vi "TimeAlign.vi"(8 "error in (no error)":errorcluster, 11 "AllData In":T1 {"FlukeData"."DataAnalysisArray"."TimeStamp" format="%^<%.3X\n%x>T"; "FlukeData"."ModelDataArray"."FREQUENCY" format="%#_6f"; "FlukeData"."ModelDataArray"."TimeStamp" format="%^<%.3X\n%x>T"; "FlukeData"."PMUDataArray"."FREQUENCY" format="%#_6f"; "FlukeData"."PMUDataArray"."TimeStamp" format="%^<%.3X\n%x>T"; "NISTData"."DataAnlysisArray"."Time" format="%.6f"; "NISTData"."DataAnlysisArray"."TimeStamp" format="%^<%.3X\n%x>T"; "NISTData"."DUTDataArray"."TimeStamp" format="%^<%.3X\n%x>T"; "NISTData"."DUTDataArray"."Time" format="%.6f"; "NISTData"."NIDataArray"."TimeStamp" format="%^<%.3X\n%x>T"; "NISTData"."NIDataArray"."Time" format="%.6f"}) -> (0 "error out":errorcluster, 3 "AllData Out":T1 {"FlukeData"."DataAnalysisArray"."TimeStamp" format="%^<%.3X\n%x>T"; "FlukeData"."ModelDataArray"."FREQUENCY" format="%#_6f"; "FlukeData"."ModelDataArray"."TimeStamp" format="%^<%.3X\n%x>T"; "FlukeData"."PMUDataArray"."FREQUENCY" format="%#_6f"; "FlukeData"."PMUDataArray"."TimeStamp" format="%^<%.3X\n%x>T"; "NISTData"."DataAnlysisArray"."Time" format="%.6f"; "NISTData"."DataAnlysisArray"."TimeStamp" format="%^<%.3X\n%x>T"; "NISTData"."DUTDataArray"."TimeStamp" format="%^<%.3X\n%x>T"; "NISTData"."DUTDataArray"."Time" format="%.6f"; "NISTData"."NIDataArray"."TimeStamp" format="%^<%.3X\n%x>T"; "NISTData"."NIDataArray"."Time" format="%.6f"})   [LabVIEW 2014]
uses:
  typedefs/Alldata.ctl
  typedefs/NISTData.ctl
  typedefs/NIDataArray.ctl
  typedefs/NIData.ctl
  typedefs/PhasorRectangular.ctl
  typedefs/DUTData.ctl
  typedefs/NICalcAnalysis.ctl
  typedefs/CalcPhasorError.ctl
  typedefs/PlotDataArrays.ctl
  typedefs/PmuRawDataCluster.ctl
  typedefs/CalcAnalysis.ctl
panel:
  out "Search":timestamp
  out "Next":timestamp
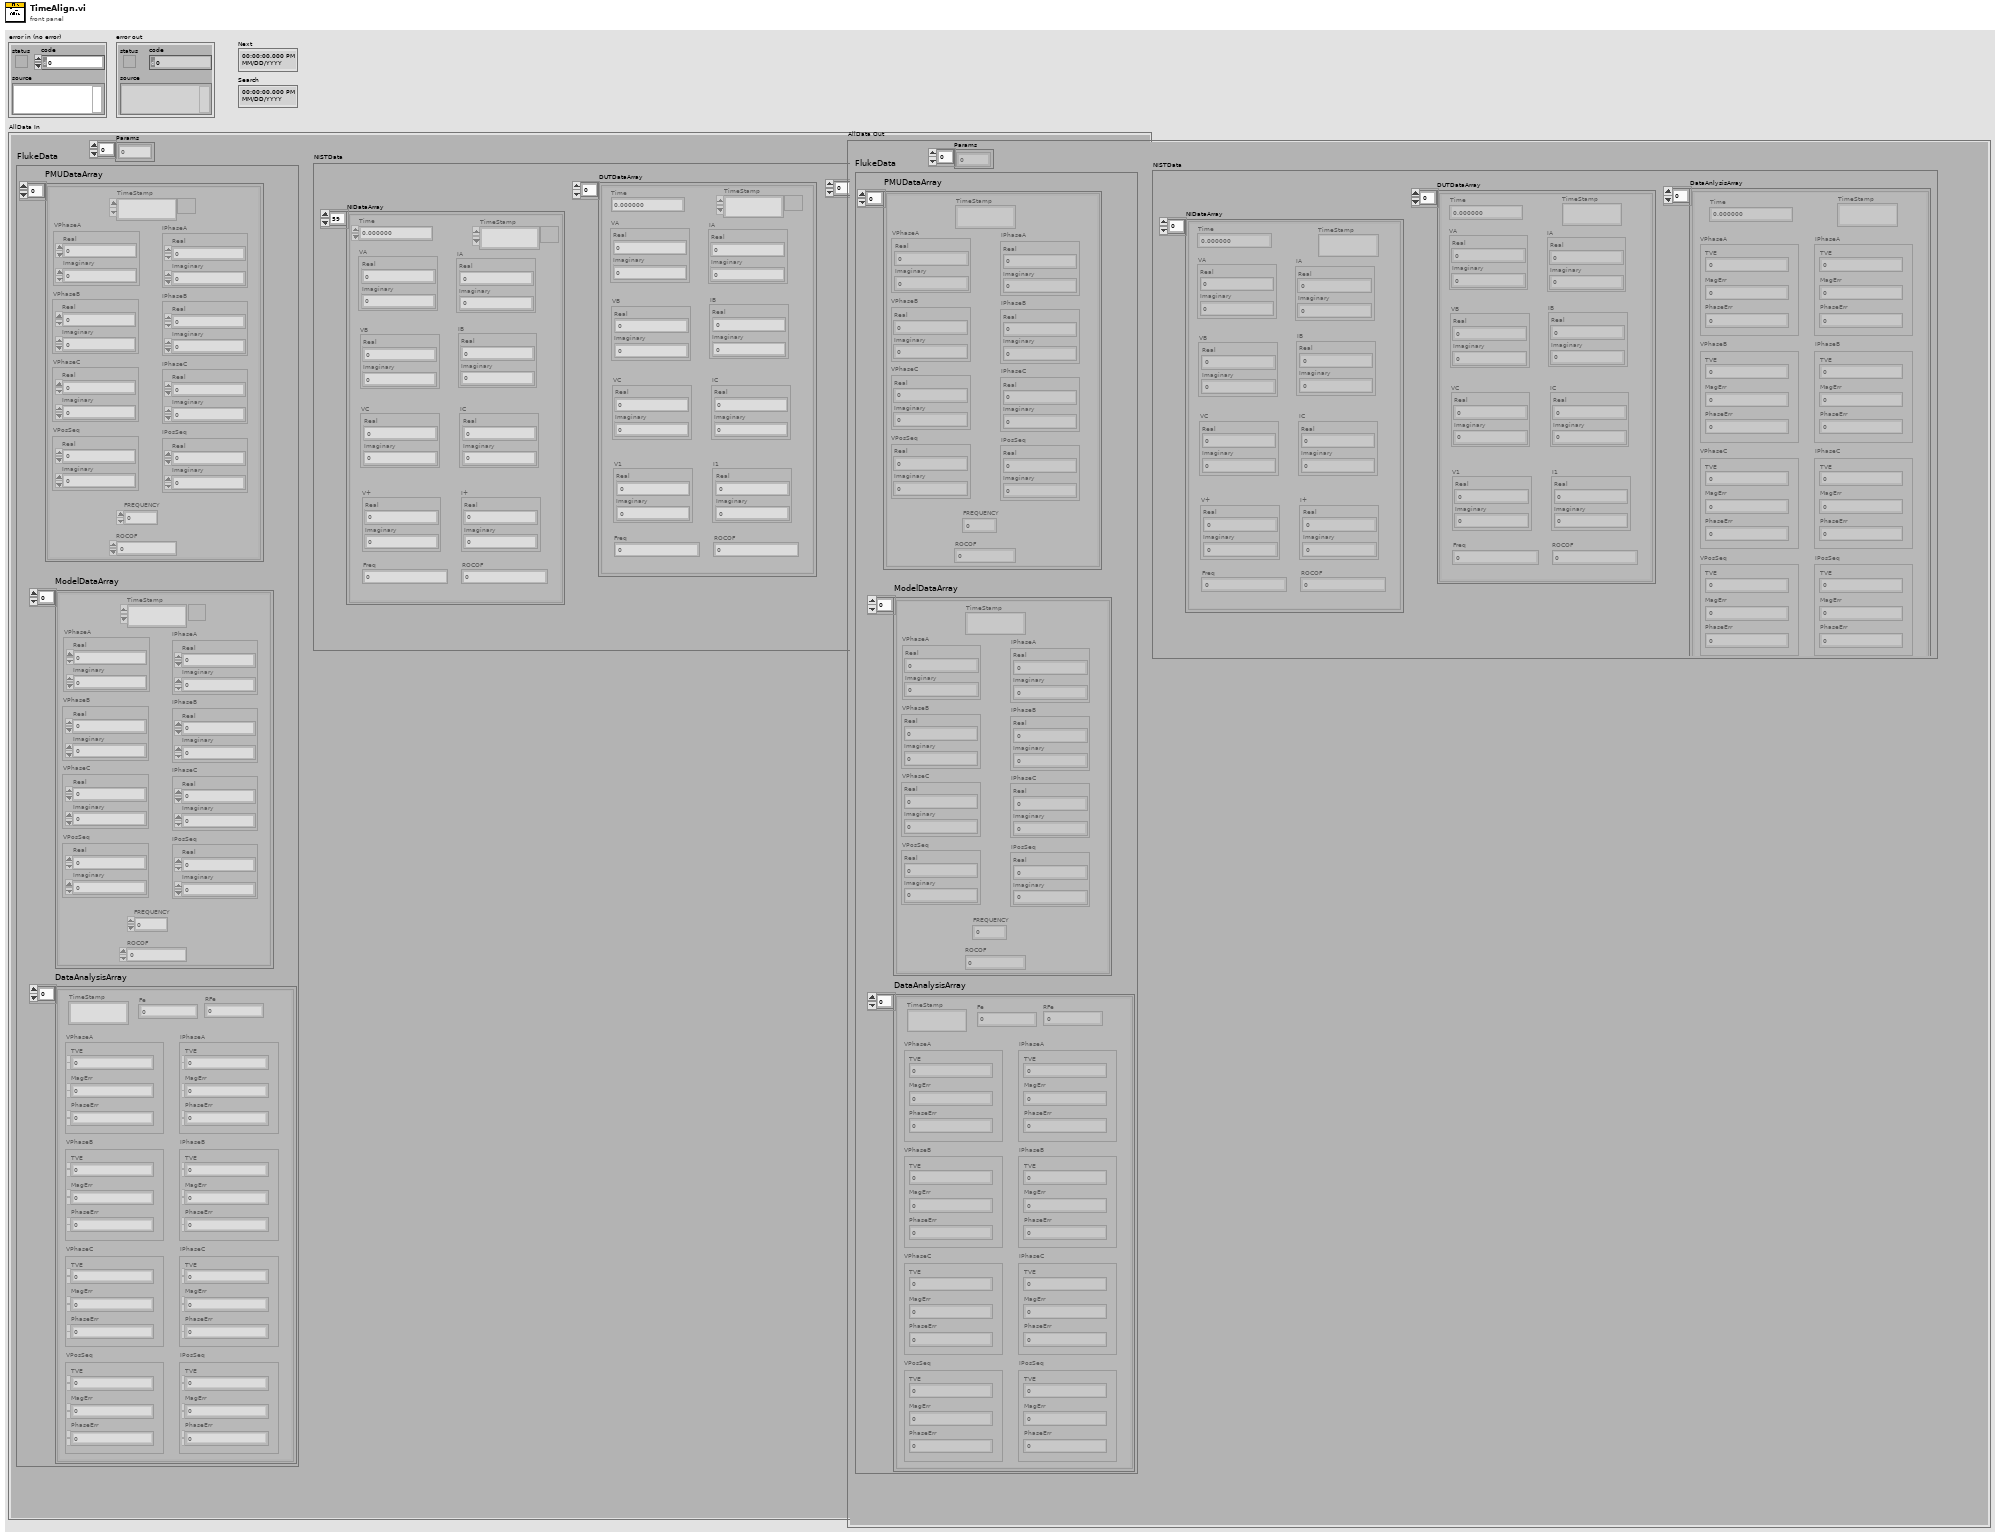
[diagram p1: front panel]
types:
  T1 = typedef "Alldata.ctl" = cluster{"NISTData":T2, "FlukeData":T9, "Params":dbl[]}
  T2 = typedef "NISTData.ctl" = cluster{"NIDataArray":T3, "DUTDataArray":T6[], "DataAnlysisArray":T7[]}
  T3 = typedef "NIDataArray.ctl" = T4[]
  T4 = typedef "NIData.ctl" = cluster{"Time":dbl, "VA":T5, "VB":T5, "VC":T5, "V+":T5, "IA":T5, "IB":T5, "IC":T5, "I+":T5, "Freq":dbl, "ROCOF":dbl, "TimeStamp":timestamp}
  T5 = typedef "PhasorRectangular.ctl" = cluster{"Real":dbl, "Imaginary":dbl}
  T6 = typedef "DUTData.ctl" = cluster{"Time":dbl, "VA":T5, "VB":T5, "VC":T5, "V1":T5, "IA":T5, "IB":T5, "IC":T5, "I1":T5, "Freq":dbl, "ROCOF":dbl, "TimeStamp":timestamp}
  T7 = typedef "NICalcAnalysis.ctl" = cluster{"Time":dbl, "VPhaseA":T8, "VPhaseB":T8, "VPhaseC":T8, "VPosSeq":T8, "IPhaseA":T8, "IPhaseB":T8, "IPhaseC":T8, "IPosSeq":T8, "Fe":dbl, "RFe":dbl, "TimeStamp":timestamp}
  T8 = typedef "CalcPhasorError.ctl" = cluster{"TVE":dbl, "MagErr":dbl, "PhaseErr":dbl}
  T9 = typedef "PlotDataArrays.ctl" = cluster{"PMUDataArray":T10[], "ModelDataArray":T10[], "DataAnalysisArray":T11[]}
  T10 = typedef "PmuRawDataCluster.ctl" = cluster{"TimeStamp":timestamp, "VPhaseA":T5, "VPhaseB":T5, "VPhaseC":T5, "VPosSeq":T5, "IPhaseA":T5, "IPhaseB":T5, "IPhaseC":T5, "IPosSeq":T5, "FREQUENCY":dbl, "ROCOF":sgl}
  T11 = typedef "CalcAnalysis.ctl" = cluster{"TimeStamp":timestamp, "VPhaseA":T8, "VPhaseB":T8, "VPhaseC":T8, "VPosSeq":T8, "IPhaseA":T8, "IPhaseB":T8, "IPhaseC":T8, "IPosSeq":T8, "Fe":dbl, "RFe":dbl}
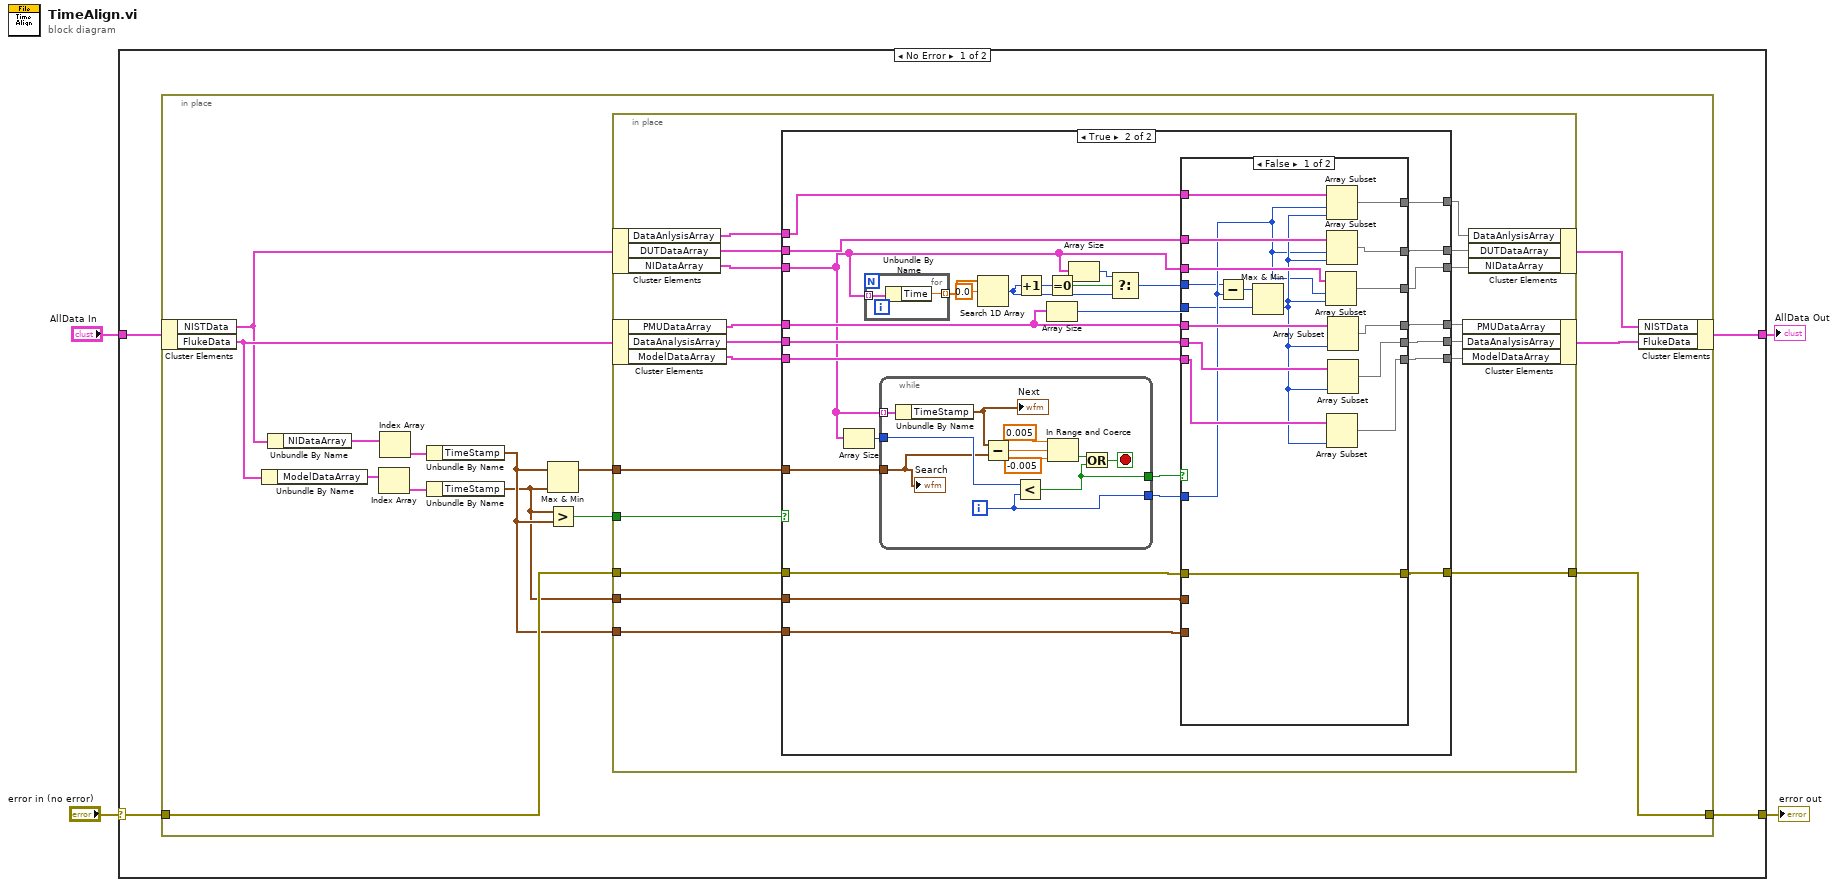
[diagram p0: block diagram]
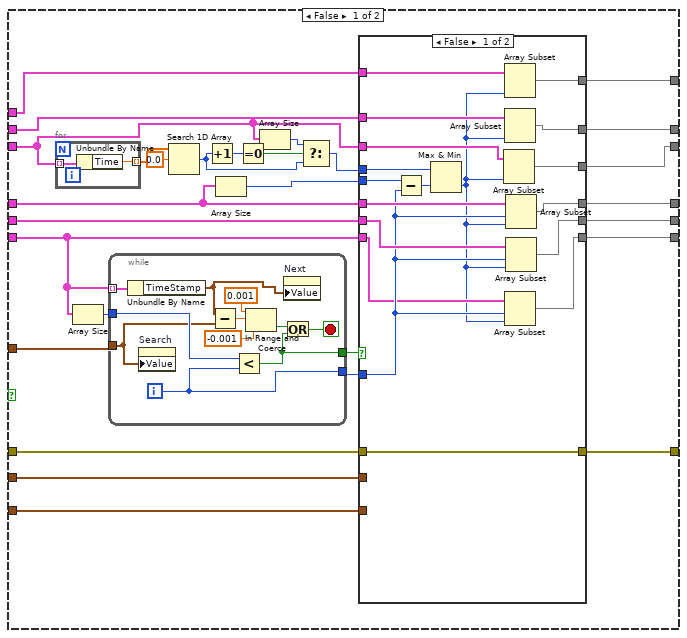
[diagram p2: hidden frame]
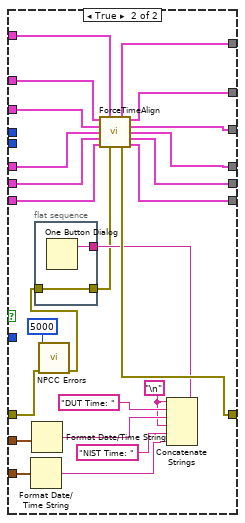
[diagram p3: hidden frame]
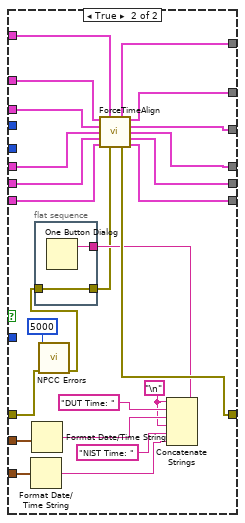
[diagram p4: hidden frame]
diagram:
  n1 = case shown="No Error" "error in (no error)" {
    selector: "error in (no error)" -> [w5 w214]
    tunnel: [w6 w214] -> w3
    tunnel: "AllData In" -> [w8 w213]
    tunnel: [w7 w213] -> w1
    frame No Error {
      n2 = in-place {
        in-place-border: [w12] -> w6
        in-place-border: w5 -> [w13]
        n3 = in-place-cluster #1(w8) -> ("NISTData"=w11:T2, "FlukeData"=w18:T9)
        n4 = Unbundle By Name(w18) -> ("ModelDataArray"=w21:T10[])
        n5 = Unbundle By Name(w11) -> ("NIDataArray"=w22:T3)
        n6 = Index Array(array=w21) -> (element=w20:T10)  [unwired: 1 in]
        n7 = Index Array(array=w22) -> (element=w19:T4)  [unwired: 1 in]
        n8 = Unbundle By Name(w19) -> ("TimeStamp"=w10:timestamp)
        n9 = Unbundle By Name(w20) -> ("TimeStamp"=w9:timestamp)
        n10 = Max & Min(x=w10, y=w9) -> (max(x,y)=w14:timestamp)  [unwired: 1 out]
        n11 = Greater?(x=w9, y=w10) -> (0:w15:bool)
        n12 = in-place {
          in-place-border: w15 -> [w40]
          in-place-border: w14 -> [w36]
          in-place-border: w13 -> [w28]
          in-place-border: [w27] -> w12
          in-place-border: w10 -> [w24]
          in-place-border: w9 -> [w23]
          n13 = in-place-cluster #2(w11) -> ("DataAnlysisArray"=w26:T7[], "DUTDataArray"=w35:T6[], "NIDataArray"=w34:T3)
          n14 = in-place-cluster #3(w18) -> ("PMUDataArray"=w39:T10[], "DataAnalysisArray"=w38:T11[], "ModelDataArray"=w37:T10[])
          n15 = case shown="True" w40 {
            tunnel: w39 -> [w63 w149]
            tunnel: w38 -> [w67 w148]
            tunnel: w37 -> [w57 w147]
            tunnel: w36 -> [w68 w154]
            tunnel: w35 -> [w60 w151]
            tunnel: w34 -> [w42 w131]
            tunnel: [w59 w140] -> w33
            tunnel: [w58 w138] -> w32
            tunnel: [w66 w139] -> w31
            tunnel: [w65 w137] -> w30
            tunnel: [w64 w136] -> w29
            tunnel: w28 -> [w54 w144]
            tunnel: [w53 w135] -> w27
            tunnel: w26 -> [w52 w152]
            tunnel: [w51 w141] -> w25
            tunnel: w24 -> [w50 w142]
            tunnel: w23 -> [w49 w143]
            frame False {
              n16 = for {
                tunnel: w42 -> [w70] mode=indexing
                tunnel: [w69] -> w47 mode=indexing
                n17 = Unbundle By Name(w70) -> ("Time"=w69:dbl)
              }
              n18 = Array Size(array=w57) -> (size(s)=w56:i32)
              n19 = while {
                tunnel: w57 -> [w126] mode=indexing
                tunnel: w68 -> [w116]
                tunnel: [w125] -> w62
                tunnel: w56 -> [w124]
                tunnel: [w122] -> w55
                i -> [w125]
                stop <- w123 stop-if-true
                n20 = Unbundle By Name(w126) -> ("TimeStamp"=w117:timestamp)
                n21 = property on="Search" class="AbsTime (strict)"("Value"=w116) -> ()  [unwired: 2 in, 2 out]
                n22 = Subtract(x=w117, y=w116) -> (x-y=w121:dbl)
                n23 = Less?(x=w124, y=w125) -> (x < y?=w122:bool)
                n24 = In Range and Coerce(upper limit=0.001, x=w121, lower limit=-0.001 ("upper limit")) -> (In Range?=w118:bool)  [unwired: 1 out]
                n25 = Or(x=w118, y=w122) -> (x .or. y?=w123:bool)
                n26 = property on="Next" class="AbsTime (strict)"("Value"=w117) -> ()  [unwired: 2 in, 2 out]
              }
              n27 = Search 1D Array(1D array=w47, element=0.0) -> (index of element=w41:i32)  [unwired: 1 in]
              n28 = Increment(x=w41) -> (x+1=w48:i32)
              n29 = Array Size(array=w63) -> (size(s)=w61:i32)
              n30 = Equal To 0?(x=w48) -> (x = 0?=w45:bool)
              n31 = Array Size(array=w42) -> (size(s)=w44:i32)
              n32 = Select(t=w44, s=w45, f=w41) -> (s? t:f=w43:i32)
              n33 = case shown="False" w55 {
                tunnel: w67 -> [w88 w102]
                tunnel: [w87 w103] -> w66
                tunnel: [w86 w104] -> w65
                tunnel: [w85 w105] -> w64
                tunnel: w63 -> [w84 w101]
                tunnel: w62 -> [w83 _]
                tunnel: w61 -> [w82 _]
                tunnel: w43 -> [w80 _]
                tunnel: w60 -> [w79 w110]
                tunnel: w42 -> [w78 w107]
                tunnel: [w77 w109] -> w59
                tunnel: [w76 w108] -> w58
                tunnel: w57 -> [w75 w106]
                tunnel: w54 -> [w74 w93]
                tunnel: [w74 w113] -> w53
                tunnel: w52 -> [w72 w112]
                tunnel: [w71 w111] -> w51
                tunnel: w50 -> [_ w100]
                tunnel: w49 -> [_ w99]
                frame False {
                  n34 = Subtract(x=w82, y=w83) -> (x-y=w81:i32)
                  n35 = Max & Min(x=w80, y=w81) -> (min(x,y)=w73:i32)  [unwired: 1 out]
                  n36 = Array Subset(array=w78, length=w73) -> (w76:T3)  [unwired: 1 in]
                  n37 = Array Subset(array=w72, length=w73) -> (w71:T7[])  [unwired: 1 in]
                  n38 = Array Subset(array=w79, length=w73) -> (w77:T6[])  [unwired: 1 in]
                  n39 = Array Subset(array=w75, index=w83, length=w73) -> (w85:T10[])
                  n40 = Array Subset(array=w84, index=w83, length=w73) -> (w87:T10[])
                  n41 = Array Subset(array=w88, index=w83, length=w73) -> (w86:T11[])
                }
                frame True {
                  w94 = "\n"
                  n42 = Format Date/Time String(seconds (now)=w100) -> (date/time string=w95:string)  [unwired: 2 in]
                  n43 = Format Date/Time String(seconds (now)=w99) -> (date/time string=w97:string)  [unwired: 2 in]
                  n44 = flat-sequence {
                    tunnel: w91 -> [w115]
                    tunnel: w90 -> [w114]
                    tunnel: [w114] -> w89
                    frame #0 {
                      n45 = One Button Dialog(message=w115) -> ()  [unwired: 1 in, 1 out]
                    }
                  }
                  n46 = call "NPCC Errors.vi"("error in (no error)"=w93, "[error code] (0)"=5000) -> ("error out"=w90:errorcluster)  [unwired: 9 in]
                  n47 = call "ForceTimeAlign.vi"("DUTDataArray"=w110, "NIAnalysisArray"=w112, "NIDataArray"=w107, "PMUDataArray"=w101, "DataAnalysisArray"=w102, "ModelDataArray"=w106, "error in (no error)"=w89) -> ("NIAnalysisArray 2"=w111:T7[], "DUTDataArray"=w109:T6[], "NIDataArray"=w108:T3, "PMUDataArray"=w103:T10[], "DataAnalysisArray"=w104:T11[], "error out"=w113:errorcluster, "ModelDataArray"=w105:T10[])  [unwired: 2 in]
                  n48 = Concatenate Strings(w94, "DUT Time: ", w97, w94, "NIST Time: ", w95) -> (w91:string)
                }
              }
            }
            frame True {
              n49 = Array Size(array=w131) -> (size(s)=w153:i32)
              n50 = for {
                tunnel: w131 -> [w156] mode=indexing
                tunnel: [w155] -> w134 mode=indexing
                n51 = Unbundle By Name(w156) -> ("Time"=w155:dbl)
              }
              n52 = while {
                tunnel: w131 -> [w212] mode=indexing
                tunnel: w154 -> [w207]
                tunnel: [w202] -> w145
                tunnel: w153 -> [w211]
                tunnel: [w209] -> w146
                i -> [w202]
                stop <- w210 stop-if-true
                n53 = Unbundle By Name(w212) -> ("TimeStamp"=w208:timestamp)
                "Next" <- w208
                n54 = Subtract(x=w208, y=w207) -> (x-y=w206:dbl)
                n55 = Less?(x=w211, y=w202) -> (x < y?=w209:bool)
                n56 = In Range and Coerce(upper limit=0.005, x=w206, lower limit=-0.005 ("upper limit")) -> (In Range?=w204:bool)  [unwired: 1 out]
                n57 = Or(x=w204, y=w209) -> (x .or. y?=w210:bool)
                "Search" <- w207
              }
              n58 = Search 1D Array(1D array=w134, element=0.0) -> (index of element=w127:i32)  [unwired: 1 in]
              n59 = Increment(x=w127) -> (x+1=w128:i32)
              n60 = Equal To 0?(x=w128) -> (x = 0?=w132:bool)
              n61 = Array Size(array=w149) -> (size(s)=w150:i32)
              n62 = Array Size(array=w131) -> (size(s)=w130:i32)
              n63 = Select(t=w130, s=w132, f=w127) -> (s? t:f=w129:i32)
              n64 = case shown="False" w146 {
                tunnel: w148 -> [w174 w188]
                tunnel: [w173 w189] -> w139
                tunnel: [w172 w190] -> w137
                tunnel: [w171 w191] -> w136
                tunnel: w149 -> [w170 w187]
                tunnel: w145 -> [w160 _]
                tunnel: w150 -> [w157 _]
                tunnel: w129 -> [w159 _]
                tunnel: w151 -> [w169 w196]
                tunnel: w131 -> [w168 w193]
                tunnel: [w167 w195] -> w140
                tunnel: [w166 w194] -> w138
                tunnel: w147 -> [w165 w192]
                tunnel: w144 -> [w164 w179]
                tunnel: [w164 w199] -> w135
                tunnel: w152 -> [w162 w198]
                tunnel: [w161 w197] -> w141
                tunnel: w142 -> [_ w186]
                tunnel: w143 -> [_ w185]
                frame False {
                  n65 = Subtract(x=w159, y=w160) -> (x-y=w158:i32)
                  n66 = Max & Min(x=w158, y=w157) -> (min(x,y)=w163:i32)  [unwired: 1 out]
                  n67 = Array Subset(array=w168, index=w160, length=w163) -> (w166:T3)
                  n68 = Array Subset(array=w162, index=w160, length=w163) -> (w161:T7[])
                  n69 = Array Subset(array=w169, index=w160, length=w163) -> (w167:T6[])
                  n70 = Array Subset(array=w165, length=w163) -> (w171:T10[])  [unwired: 1 in]
                  n71 = Array Subset(array=w170, length=w163) -> (w173:T10[])  [unwired: 1 in]
                  n72 = Array Subset(array=w174, length=w163) -> (w172:T11[])  [unwired: 1 in]
                }
                frame True {
                  w180 = "\n"
                  n73 = Format Date/Time String(seconds (now)=w186) -> (date/time string=w181:string)  [unwired: 2 in]
                  n74 = Format Date/Time String(seconds (now)=w185) -> (date/time string=w183:string)  [unwired: 2 in]
                  n75 = flat-sequence {
                    tunnel: w177 -> [w201]
                    tunnel: w176 -> [w200]
                    tunnel: [w200] -> w175
                    frame #0 {
                      n76 = One Button Dialog(message=w201) -> ()  [unwired: 1 in, 1 out]
                    }
                  }
                  n77 = call "NPCC Errors.vi"("error in (no error)"=w179, "[error code] (0)"=5000) -> ("error out"=w176:errorcluster)  [unwired: 9 in]
                  n78 = call "ForceTimeAlign.vi"("DUTDataArray"=w196, "NIAnalysisArray"=w198, "NIDataArray"=w193, "PMUDataArray"=w187, "DataAnalysisArray"=w188, "ModelDataArray"=w192, "error in (no error)"=w175) -> ("NIAnalysisArray 2"=w197:T7[], "DUTDataArray"=w195:T6[], "NIDataArray"=w194:T3, "PMUDataArray"=w189:T10[], "DataAnalysisArray"=w190:T11[], "error out"=w199:errorcluster, "ModelDataArray"=w191:T10[])  [unwired: 2 in]
                  n79 = Concatenate Strings(w180, "DUT Time: ", w183, w180, "NIST Time: ", w181) -> (w177:string)
                }
              }
            }
          }
          n80 = in-place-cluster #3("PMUDataArray"=w31, "DataAnalysisArray"=w30, "ModelDataArray"=w29) -> (w17:T9)
          n81 = in-place-cluster #2("DataAnlysisArray"=w25, "DUTDataArray"=w33, "NIDataArray"=w32) -> (w16:T2)
        }
        n82 = in-place-cluster #1("NISTData"=w16, "FlukeData"=w17) -> (w7:T1)
      }
    }
    frame Error {
    }
  }
  "error out" <- w3
  "AllData Out" <- w1
